vi "Seq Dialog Set or Check String.vi"(8 "Segment Data":T1) -> (0 "Step Hisitory":string[](array[string]), 2 "Segment Data 2":T1)   [LabVIEW 2018]
uses:
  type defs/Sequence Info.ctl
panel:
  in  "String":string
  out "String 2":string="Pre Run Station - Glass - Vent Open"
  in  "Description":string
  in  "Save":bool
  in  "Cancel":bool
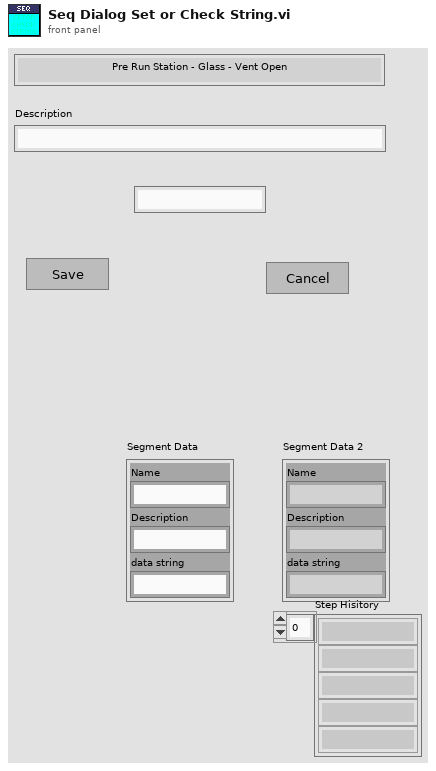
[diagram p1: front panel]
types:
  T1 = typedef "Sequence Info.ctl" = cluster{"Name":string, "Description":string, "data string":string}
  T2 = cluster{"Segment Data":T1, "Old Data":string, "New Data":string}
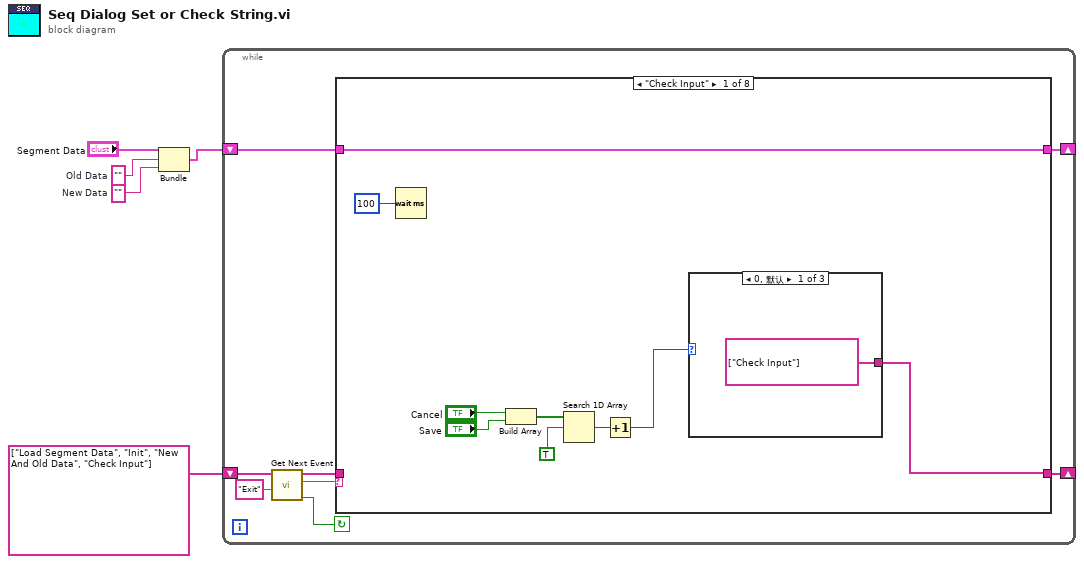
[diagram p0: block diagram]
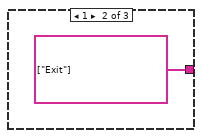
[diagram p2: hidden frame]
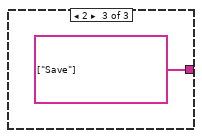
[diagram p3: hidden frame]
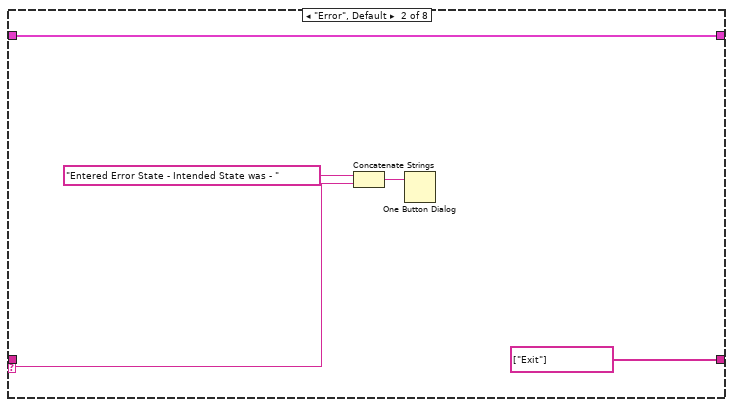
[diagram p4: hidden frame]
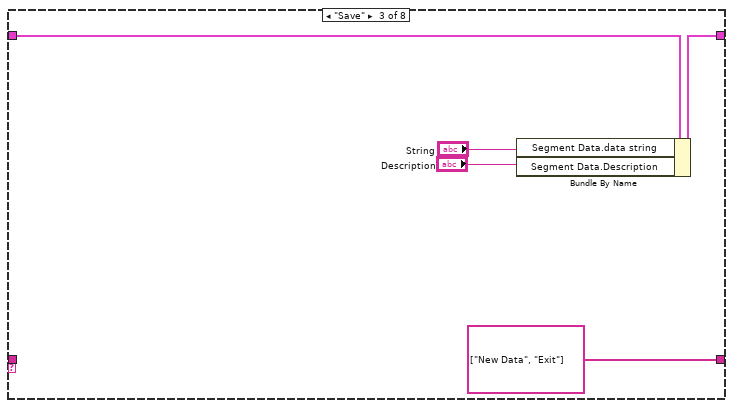
[diagram p5: hidden frame]
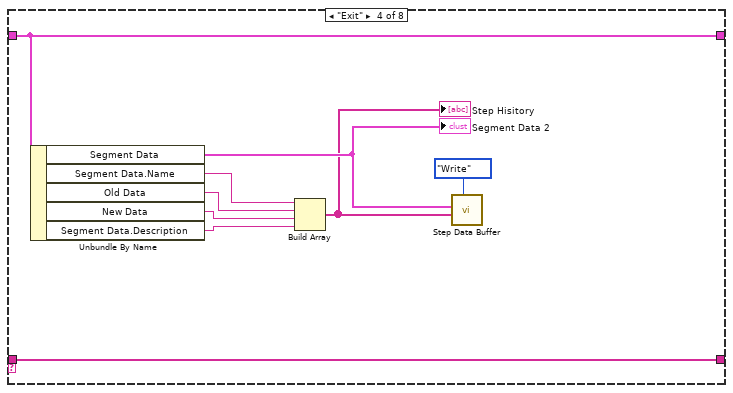
[diagram p6: hidden frame]
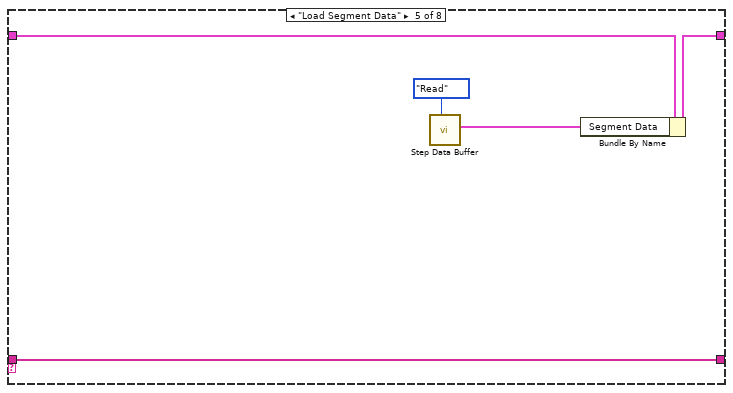
[diagram p7: hidden frame]
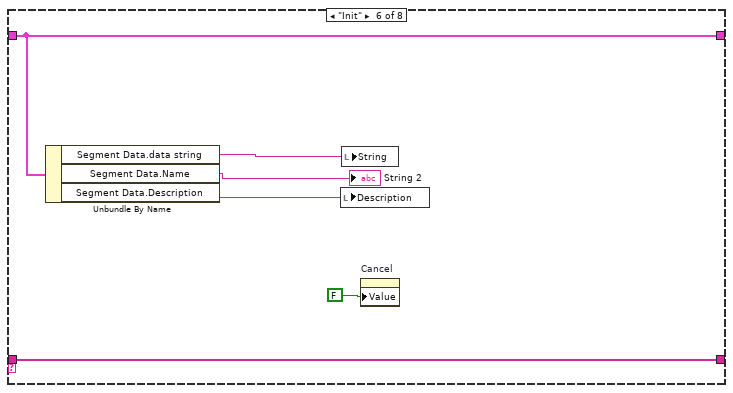
[diagram p8: hidden frame]
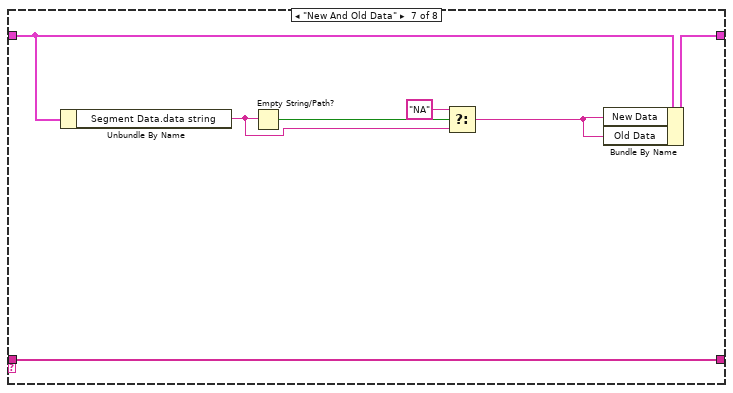
[diagram p9: hidden frame]
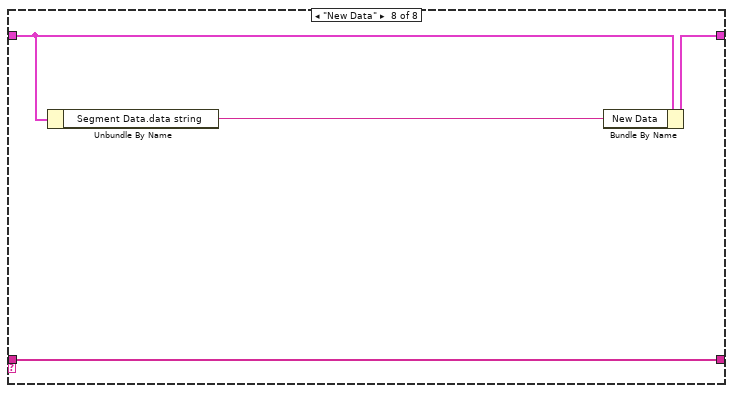
[diagram p10: hidden frame]
diagram:
  w3 = ""  # New Data
  w4 = ""  # Old Data
  n1 = Bundle("Segment Data"="Segment Data", "Old Data"=w4, "New Data"=w3) -> (w1:T2)  [unwired: 1 in]
  n2 = while {
    shift-right: [w11] -> _
    shift-left: string[] ["Load Segment Data", "Init", "New And Old Data", "Check Input"] ("Event queue out") -> [w10]
    shift-right: [w6] -> _
    shift-left: w1 -> [w7]
    stop <- w9 continue-if-true
    n3 = call "Get Next Event.vi"("Exit Event"="Exit", "event queue in"=w10) -> ("Condition (Exit:F)"=w9:bool, "next event"=w13:string, "event queue out"=w12:string[])  [unwired: 3 in]
    n4 = case shown="\"Check Input\"" w13 {
      selector: w13 -> [_ w26 _ _ _ _ _ _]
      tunnel: w12 -> [_ _ _ w44 w49 w55 w62 w66]
      tunnel: [w14 string[] ["Exit"] ("event queue out") string[] ["New Data", "Exit"] ("Event queue out") w44 w49 w55 w62 w66] -> w11
      tunnel: w7 -> [w17 w30 w32 w40 w48 w51 w61 w65]
      tunnel: [w17 w30 w34 w40 w46 w51 w60 w64] -> w6
      frame "Check Input" {
        n5 = Wait (ms)(milliseconds to wait=u32 100) -> ()  [unwired: 1 out]
        n6 = Build Array("Cancel", "Save") -> (w19:bool[])
        n7 = Search 1D Array(1D array=w19, element=TRUE) -> (index of element=w16:i32)  [unwired: 1 in]
        n8 = Increment(x=w16) -> (x+1=w15:i32)
        n9 = case shown="0, 默认" w15 {
          tunnel: [string[] ["Check Input"] ("Events to Insert") string[] ["Exit"] ("Events to Insert") string[] ["Save"] ("Events to Insert")] -> w14
          frame 0, Default {
          }
          frame 1 {
          }
          frame 2 {
          }
        }
      }
      frame "Error", Default {
        n10 = Concatenate Strings("Entered Error State - Intended State was - " ("string"), w26) -> (w28:string)
        n11 = One Button Dialog(message=w28) -> ()  [unwired: 1 in, 1 out]
      }
      frame "Save" {
        n12 = Bundle By Name(cluster=w32, "Segment Data.data string"="String", "Segment Data.Description"="Description") -> (w34:T2)
      }
      frame "Exit" {
        n13 = Unbundle By Name(w40) -> ("Segment Data"=w38:T1, "Segment Data.Name"=w42:string, "Old Data"=w41:string, "New Data"=w43:string, "Segment Data.Description"=w36:string)
        "Segment Data 2" <- w38
        n14 = Build Array(w42, w41, w43, w36) -> (w37:string[])
        "Step Hisitory" <- w37
        n15 = call "Step Data Buffer.vi"("Mode"=enum16{"Init", "Read", "Write"}."Write", "Step Hisitory In"=w37, "Segment Data In"=w38) -> ()  [unwired: 4 in, 5 out]
      }
      frame "Load Segment Data" {
        n16 = call "Step Data Buffer.vi"("Mode"=enum16{"Init", "Read", "Write"}."Read") -> ("Segment Data Out"=w45:T1)  [unwired: 6 in, 4 out]
        n17 = Bundle By Name(cluster=w48, "Segment Data"=w45) -> (w46:T2)
      }
      frame "Init" {
        n18 = Unbundle By Name(w51) -> ("Segment Data.data string"=w52:string, "Segment Data.Name"=→"String 2":string, "Segment Data.Description"=w53:string)
        n19 = local write "Description"(w53) -> ()
        n20 = local write "String"(w52) -> ()
        n21 = property on="Cancel" class="Bool (严格)"("Value"=FALSE ("Cancel")) -> ()  [unwired: 2 in, 2 out]
      }
      frame "New And Old Data" {
        n22 = Unbundle By Name(w61) -> ("Segment Data.data string"=w56:string)
        n23 = Empty String/Path?(string/path=w56) -> (empty?=w59:bool)
        n24 = Select(t="NA", s=w59, f=w56) -> (s? t:f=w57:string)
        n25 = Bundle By Name(cluster=w61, "New Data"=w57, "Old Data"=w57) -> (w60:T2)
      }
      frame "New Data" {
        n26 = Unbundle By Name(w65) -> ("Segment Data.data string"=w63:string)
        n27 = Bundle By Name(cluster=w65, "New Data"=w63) -> (w64:T2)
      }
    }
  }
